vi "Flush Message Queue_sushu.vi"(0 "Queue In":cluster{"Q":T1, "Name":string}, 11 "error in":errorcluster) -> (4 "Queue Out":cluster{"Q":T1, "Name":string}, 6 "remaining messages":T2[](array[typedef]), 15 "error out":errorcluster)   [LabVIEW 2021]
doc: "Removes and returns all messages currently in the message queue."
uses:
  <vilib>/NI/AMC/Message.ctl
  <vilib>/NI/Tools/Keyed Array/KeyedArray.ctl
  <vilib>/NI/AMC/Message Queue.ctl
  <vilib>/NI/AMC/AMC.lvlib
  <vilib>/NI/Tools/Keyed Array/Tools_KeyedArray.lvlib
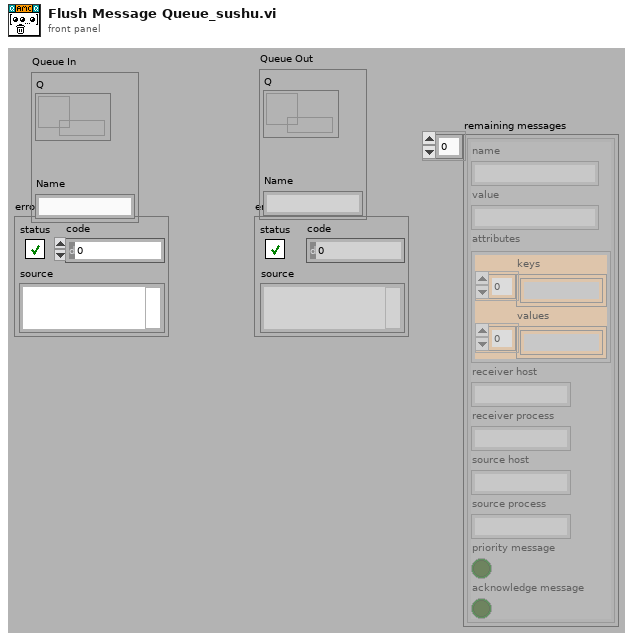
[diagram p1: front panel]
types:
  T1 = typedef "AMC.lvlib/Message Queue.ctl" = refnum<queue>
  T2 = typedef "AMC.lvlib/Message.ctl" = cluster{"name":string, "value":string, "attributes":T3, "receiver host":string, "receiver process":string, "source host":string, "source process":string, "priority message":bool, "acknowledge message":bool}
  T3 = typedef "Tools_KeyedArray.lvlib/KeyedArray.ctl" = cluster{"keys":string[], "values":string[]}
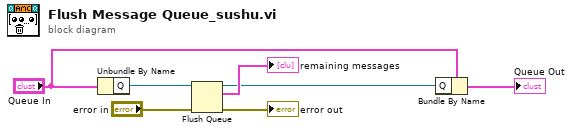
[diagram p0: block diagram]
diagram:
  n1 = Unbundle By Name("Queue In") -> ("Q"=w4:T1)
  n2 = Flush Queue(queue=w4, error in (no error)="error in") -> (queue out=w3:T1, remaining elements=→"remaining messages":T2[], error out=→"error out":errorcluster)
  n3 = Bundle By Name(cluster="Queue In", "Q"=w3) -> (→"Queue Out":cluster{"Q":T1, "Name":string})
